vi "Angle Wheels.vi"() -> ()   [LabVIEW 2018]
panel:
  in  "Angle":dbl
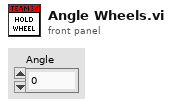
[diagram p1: front panel]
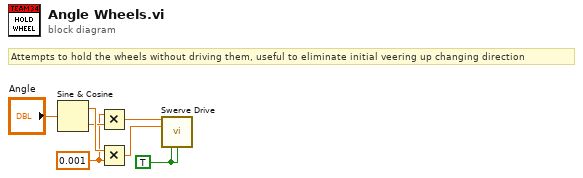
[diagram p0: block diagram]
diagram:
  w3 = TRUE ("Robot Centric?")
  w4 = 0.001 ("y")
  # "Attempts to hold the wheels without driving them, useful to eliminate initial veering up changing direction"
  n1 = Sine & Cosine(0:"Angle") -> (1:w6:dbl, 2:w5:dbl)
  n2 = Multiply(x=w4, y=w5) -> (x*y=w2:dbl)
  n3 = Multiply(x=w6, y=w4) -> (x*y=w1:dbl)
  n4 = call "Swerve Drive.vi"("X"=w2, "Y"=w1, "Robot Centric?"=w3, "Autonomous?"=w3) -> ()  [unwired: 7 in, 5 out]
